vi "CC SubSystem Message.vi"(8 "error in (no error)":errorcluster, 10 "Subsystem":string, 11 "Message":string) -> (0 "error out":errorcluster)   [LabVIEW 2021]
uses:
  Subsystems/SS cluster Data Queue type.ctl
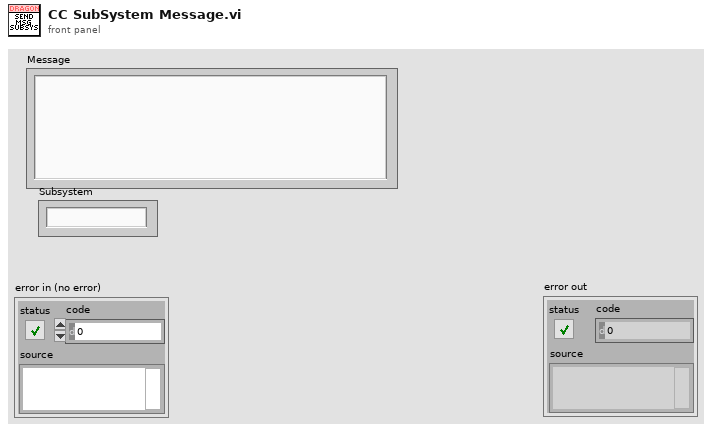
[diagram p1: front panel]
types:
  T1 = typedef "SS cluster Data Queue type.ctl" = cluster{"Source":string, "Type":string, "Data":variant}
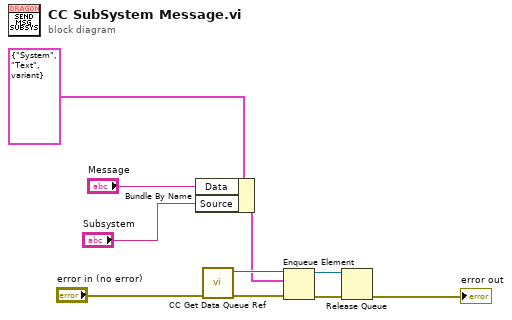
[diagram p0: block diagram]
diagram:
  n1 = Bundle By Name(cluster=T1 {"Source"="System", "Type"="Text", "Data"=variant} ("element"), "Data"="Message", "Source"="Subsystem") -> (w3:T1)
  n2 = call "CC Get Data Queue Ref.vi"("error in (no error)"="error in (no error)") -> ("error out"=w6:errorcluster, "Data Q"=w7:refnum<queue>)  [unwired: 9 in]
  n3 = Enqueue Element(queue=w7, element=w3, error in (no error)=w6) -> (queue out=w10:refnum<queue>, error out=w9:errorcluster)  [unwired: 1 in, 1 out]
  n4 = Release Queue(queue=w10, error in (no error)=w9) -> (error out=→"error out":errorcluster)  [unwired: 1 in, 2 out]
